vi "subvi_determinemove.vi"(10 "white lacation":cluster{"Numeric":i32, "Numeric 2":i32}, 11 "puzzle lacation":cluster{"Numeric":i32, "Numeric 2":i32}) -> (0 "Upper White Row Position":i32, 1 "Current Peice Column":i32, 2 "Current Peice Row":i32, 3 "Lower White Column Position":i32, 5 "Allow Peice Movement":bool)   [LabVIEW 2014]
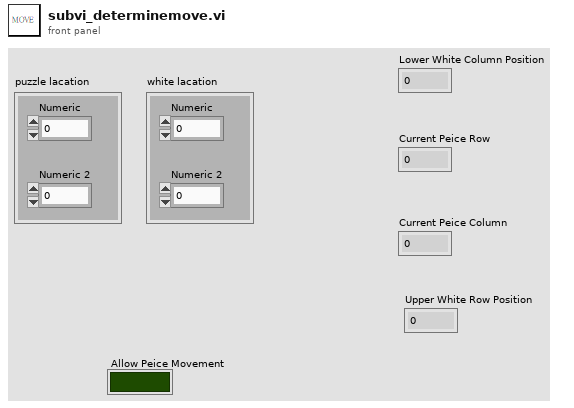
[diagram p1: front panel]
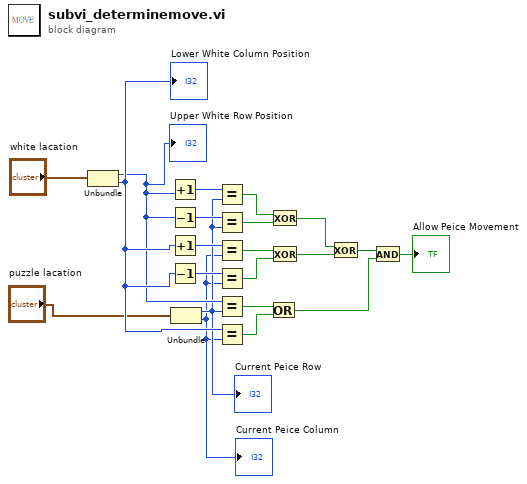
[diagram p0: block diagram]
diagram:
  n1 = Unbundle("white lacation") -> ("Numeric"=w20:i32, "Numeric 2"=w21:i32)
  "Lower White Column Position" <- w21
  "Upper White Row Position" <- w20
  n2 = Increment(x=w20) -> (x+1=w18:i32)
  n3 = Decrement(x=w20) -> (x-1=w17:i32)
  n4 = Increment(x=w21) -> (x+1=w16:i32)
  n5 = Decrement(x=w21) -> (x-1=w15:i32)
  n6 = Unbundle("puzzle lacation") -> ("Numeric"=w8:i32, "Numeric 2"=w7:i32)
  "Current Peice Column" <- w7
  "Current Peice Row" <- w8
  n7 = Equal?(x=w18, y=w8) -> (x = y?=w14:bool)
  n8 = Equal?(x=w17, y=w8) -> (x = y?=w13:bool)
  n9 = Equal?(x=w16, y=w7) -> (x = y?=w12:bool)
  n10 = Equal?(x=w15, y=w7) -> (x = y?=w11:bool)
  n11 = Equal?(x=w20, y=w8) -> (x = y?=w2:bool)
  n12 = Equal?(x=w21, y=w7) -> (x = y?=w3:bool)
  n13 = Or(x=w2, y=w3) -> (x .or. y?=w4:bool)
  n14 = Exclusive Or(1:w13, 2:w14) -> (0:w10:bool)
  n15 = Exclusive Or(1:w11, 2:w12) -> (0:w9:bool)
  n16 = Exclusive Or(1:w9, 2:w10) -> (0:w5:bool)
  n17 = And(x=w5, y=w4) -> (x .and. y?=→"Allow Peice Movement":bool)
